vi "Termination Character-Default--Const.vi"() -> (3 "Termination Character":string)   [LabVIEW 2017, in "Communications Library.lvlib"]
uses:
  Communications Library.lvlib
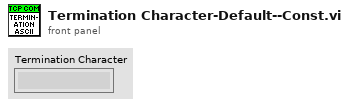
[diagram p1: front panel]
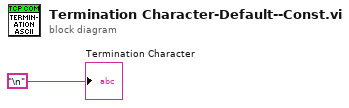
[diagram p0: block diagram]
diagram:
  "Termination Character" <- "\n"
